vi "Finish.vi"   [LabVIEW 2015]
doc: "This VI is called just before exiting. It is expected to close I/O refnum, save collected data, etc."
uses:
  SubSystems/References/Refnums.vi
  <vilib>/Rock Robotics/WPI/Utilities/WPI_GetSetVariantRefNum.vi
types:
  T1 = typedef "WPI_RelayDevRef.ctl" = cluster{"DevStatus":errorcluster, "Relay Channel":T2, "Relay Direction":T3}
  T2 = typedef "FPGA_DIORelayChannel.ctl" = enum8{"Relay 0", "Relay 1", "Relay 2", "Relay 3", "Invalid"}
  T3 = typedef "WPI_RelayDirection.ctl" = enum16{"Both directions", "Forward only", "Reverse only"}
  T4 = typedef "WPI_DigitalInputDevRef.ctl" = cluster{"DevStatus":errorcluster, "DIO Channel":T5}
  T5 = typedef "FPGA_DIOChannel.ctl" = enum8{"DIO 0", "DIO 1", "DIO 2", "DIO 3", "DIO 4", "DIO 5", "DIO 6", "DIO 7", "DIO 8", "DIO 9", "DIO MXP 0", "DIO MXP 1", "DIO MXP 2", "DIO MXP 3", "DIO MXP 4", "DIO MXP 5", "DIO MXP 6", "DIO MXP 7", "DIO MXP 8", "DIO MXP 9", "DIO MXP 10", "DIO MXP 11", "DIO MXP 12", "DIO MXP 13", "DIO MXP 14", "DIO MXP 15", "Invalid"}
  T6 = typedef "WPI_JoystickDevRef.ctl" = cluster{"Device":T7}
  T7 = typedef "WPI_JoystickDeviceEnum.ctl" = enum16{"USB 0", "USB 1", "USB 2", "USB 3", "USB 4", "USB 5"}
  T8 = typedef "WPI_MotorControlDeviceRef.ctl" = cluster{"DeviceStatus":errorcluster, "Type":T9, "PWM":cluster{"PWM Channel":T10, "DeadBand":T11}, "CAN":cluster{"Device Number":u8, "Control Mode":T12, "Semaphore":T13, "Max Vout":dbl, "TalonSRX Control Mode":T14}, "Invert":bool}
  T9 = typedef "WPI_MotorControlType.ctl" = enum16{"PWM", "CAN", "CANTalonSRX"}
  T10 = typedef "FPGA_DIOPWMChannel.ctl" = enum8{"PWM 0", "PWM 1", "PWM 2", "PWM 3", "PWM 4", "PWM 5", "PWM 6", "PWM 7", "PWM 8", "PWM 9", "PWM MXP 0", "PWM MXP 1", "PWM MXP 2", "PWM MXP 3", "PWM MXP 4", "PWM MXP 5", "PWM MXP 6", "PWM MXP 7", "PWM MXP 8", "PWM MXP 9", "Invalid"}
  T11 = typedef "WPI_PWMDeadband.ctl" = cluster{"Name":string, "maxPositivePwm":i32, "minPositivePwm":i32, "centerPwm":i32, "maxNegativePwm":i32, "minNegativePwm":i32, "angularRange":u16}
  T12 = typedef "WPI_CANJaguar_ControlMode.ctl" = enum8{"Percent VBus", "Current", "Speed", "Position", "Voltage"}
  T13 = typedef "Semaphore RefNum" = refnum<k1>
  T14 = typedef "WPI_CANTalonSRX_APIControlMode.ctl" = enum8{"Percent VBus", "Speed", "Position", "Slave", "Unchanged / Invalid", "Voltage Compensation", "Current", "Motion Profile"}
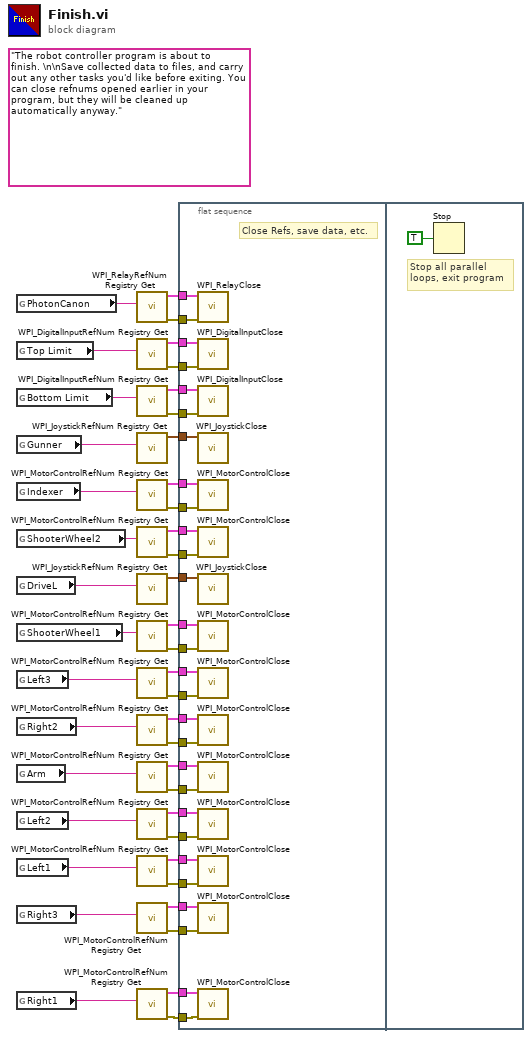
[diagram p0: block diagram]
diagram:
  (unwired) "The robot controller program is about to finish. \n\nSave collected data to files, and carry out any other tasks you'd like before exiting. You can close refnums opened earlier in your program, but they will be cleaned up automatically anyway."
  n1 = global read "Refnums.vi" "PhotonCanon"() -> (w3:string)
  n2 = global read "Refnums.vi" "Top Limit"() -> (w43:string)
  n3 = global read "Refnums.vi" "Bottom Limit"() -> (w8:string)
  n4 = global read "Refnums.vi" "Gunner"() -> (w9:string)
  n5 = global read "Refnums.vi" "Indexer"() -> (w18:string)
  n6 = global read "Refnums.vi" "ShooterWheel2"() -> (w19:string)
  n7 = global read "Refnums.vi" "DriveL"() -> (w12:string)
  n8 = global read "Refnums.vi" "ShooterWheel1"() -> (w24:string)
  n9 = global read "Refnums.vi" "Left3"() -> (w37:string)
  n10 = global read "Refnums.vi" "Right2"() -> (w41:string)
  n11 = global read "Refnums.vi" "Arm"() -> (w17:string)
  n12 = global read "Refnums.vi" "Left2"() -> (w38:string)
  n13 = global read "Refnums.vi" "Left1"() -> (w39:string)
  n14 = global read "Refnums.vi" "Right3"() -> (w40:string)
  n15 = global read "Refnums.vi" "Right1"() -> (w42:string)
  n16 = call <vilib>:"WPI_RelayRefNum Registry Get.vi"("refnum name"=w3) -> ("error out"=w1:errorcluster, "RelayDevRef"=w2:T1)  [unwired: 9 in]
  n17 = call <vilib>:"WPI_DigitalInputRefNum Registry Get.vi"("refnum name"=w43) -> ("error out"=w4:errorcluster, "DigitalInputDevRef"=w5:T4)  [unwired: 9 in]
  n18 = call <vilib>:"WPI_DigitalInputRefNum Registry Get.vi"("refnum name"=w8) -> ("error out"=w6:errorcluster, "DigitalInputDevRef"=w7:T4)  [unwired: 9 in]
  n19 = call <vilib>:"WPI_JoystickRefNum Registry Get.vi"("refnum name"=w9) -> ("JoystickDevRef"=w10:T6)  [unwired: 9 in, 1 out]
  n20 = call <vilib>:"WPI_MotorControlRefNum Registry Get.vi"("refnum name"=w18) -> ("error out"=w15:errorcluster, "MotorControlDevRef"=w16:T8)  [unwired: 9 in]
  n21 = call <vilib>:"WPI_MotorControlRefNum Registry Get.vi"("refnum name"=w19) -> ("error out"=w20:errorcluster, "MotorControlDevRef"=w21:T8)  [unwired: 9 in]
  n22 = call <vilib>:"WPI_JoystickRefNum Registry Get.vi"("refnum name"=w12) -> ("JoystickDevRef"=w11:T6)  [unwired: 9 in, 1 out]
  n23 = call <vilib>:"WPI_MotorControlRefNum Registry Get.vi"("refnum name"=w24) -> ("error out"=w22:errorcluster, "MotorControlDevRef"=w23:T8)  [unwired: 9 in]
  n24 = call <vilib>:"WPI_MotorControlRefNum Registry Get.vi"("refnum name"=w37) -> ("error out"=w25:errorcluster, "MotorControlDevRef"=w26:T8)  [unwired: 9 in]
  n25 = call <vilib>:"WPI_MotorControlRefNum Registry Get.vi"("refnum name"=w41) -> ("error out"=w33:errorcluster, "MotorControlDevRef"=w34:T8)  [unwired: 9 in]
  n26 = call <vilib>:"WPI_MotorControlRefNum Registry Get.vi"("refnum name"=w17) -> ("error out"=w13:errorcluster, "MotorControlDevRef"=w14:T8)  [unwired: 9 in]
  n27 = call <vilib>:"WPI_MotorControlRefNum Registry Get.vi"("refnum name"=w38) -> ("error out"=w27:errorcluster, "MotorControlDevRef"=w28:T8)  [unwired: 9 in]
  n28 = call <vilib>:"WPI_MotorControlRefNum Registry Get.vi"("refnum name"=w39) -> ("error out"=w29:errorcluster, "MotorControlDevRef"=w30:T8)  [unwired: 9 in]
  n29 = call <vilib>:"WPI_MotorControlRefNum Registry Get.vi"("refnum name"=w40) -> ("error out"=w31:errorcluster, "MotorControlDevRef"=w32:T8)  [unwired: 9 in]
  n30 = call <vilib>:"WPI_MotorControlRefNum Registry Get.vi"("refnum name"=w42) -> ("error out"=w35:errorcluster, "MotorControlDevRef"=w36:T8)  [unwired: 9 in]
  n31 = flat-sequence {
    tunnel: w36 -> [w71]
    tunnel: w35 -> [w70]
    tunnel: w34 -> [w69]
    tunnel: w33 -> [w68]
    tunnel: w32 -> [w67]
    tunnel: w31 -> [w66]
    tunnel: w30 -> [w65]
    tunnel: w29 -> [w64]
    tunnel: w28 -> [w63]
    tunnel: w27 -> [w62]
    tunnel: w26 -> [w61]
    tunnel: w25 -> [w60]
    tunnel: w23 -> [w59]
    tunnel: w22 -> [w58]
    tunnel: w21 -> [w57]
    tunnel: w20 -> [w56]
    tunnel: w16 -> [w55]
    tunnel: w15 -> [w54]
    tunnel: w14 -> [w53]
    tunnel: w13 -> [w52]
    tunnel: w11 -> [w51]
    tunnel: w10 -> [w50]
    tunnel: w7 -> [w49]
    tunnel: w6 -> [w48]
    tunnel: w5 -> [w47]
    tunnel: w4 -> [w46]
    tunnel: w2 -> [w45]
    tunnel: w1 -> [w44]
    frame #0 {
      # "Close Refs, save data, etc."
      n32 = call <vilib>:"WPI_RelayClose.vi"("error in (no error)"=w44, "RelayDevRef"=w45) -> ()  [unwired: 9 in, 1 out]
      n33 = call <vilib>:"WPI_DigitalInputClose.vi"("error in (no error)"=w46, "DigitalInputDevRef"=w47) -> ()  [unwired: 9 in, 1 out]
      n34 = call <vilib>:"WPI_DigitalInputClose.vi"("error in (no error)"=w48, "DigitalInputDevRef"=w49) -> ()  [unwired: 9 in, 1 out]
      n35 = call <vilib>:"WPI_JoystickClose.vi"("JoystickDevRef"=w50) -> ()  [unwired: 11 in]
      n36 = call <vilib>:"WPI_MotorControlClose.vi"("error in (no error)"=w54, "MotorControlDevRef"=w55) -> ()  [unwired: 9 in, 1 out]
      n37 = call <vilib>:"WPI_MotorControlClose.vi"("error in (no error)"=w56, "MotorControlDevRef"=w57) -> ()  [unwired: 9 in, 1 out]
      n38 = call <vilib>:"WPI_JoystickClose.vi"("JoystickDevRef"=w51) -> ()  [unwired: 11 in]
      n39 = call <vilib>:"WPI_MotorControlClose.vi"("error in (no error)"=w58, "MotorControlDevRef"=w59) -> ()  [unwired: 9 in, 1 out]
      n40 = call <vilib>:"WPI_MotorControlClose.vi"("error in (no error)"=w60, "MotorControlDevRef"=w61) -> ()  [unwired: 9 in, 1 out]
      n41 = call <vilib>:"WPI_MotorControlClose.vi"("error in (no error)"=w68, "MotorControlDevRef"=w69) -> ()  [unwired: 9 in, 1 out]
      n42 = call <vilib>:"WPI_MotorControlClose.vi"("error in (no error)"=w52, "MotorControlDevRef"=w53) -> ()  [unwired: 9 in, 1 out]
      n43 = call <vilib>:"WPI_MotorControlClose.vi"("error in (no error)"=w62, "MotorControlDevRef"=w63) -> ()  [unwired: 9 in, 1 out]
      n44 = call <vilib>:"WPI_MotorControlClose.vi"("error in (no error)"=w64, "MotorControlDevRef"=w65) -> ()  [unwired: 9 in, 1 out]
      n45 = call <vilib>:"WPI_MotorControlClose.vi"("error in (no error)"=w66, "MotorControlDevRef"=w67) -> ()  [unwired: 9 in, 1 out]
      n46 = call <vilib>:"WPI_MotorControlClose.vi"("error in (no error)"=w70, "MotorControlDevRef"=w71) -> ()  [unwired: 9 in, 1 out]
    }
    frame #1 {
      # "Stop all parallel\nloops, exit program"
      n47 = Stop(stop? (T)=TRUE ("Quit")) -> ()
    }
  }
